vi "Message Available.vi"(8 "error in":errorcluster, 11 "VISA resource name":refnum<visa-resource-name>) -> (0 "error out":errorcluster, 2 "message available":bool, 3 "VISA resource name out":refnum<visa-resource-name>)   [LabVIEW 2019, in "Andeen-Hagerling 2700(400 firmware).lvlib"]
doc: "Poll the VISA resource to check if a message is available to read."
uses:
  Andeen-Hagerling 2700(400 firmware).lvlib
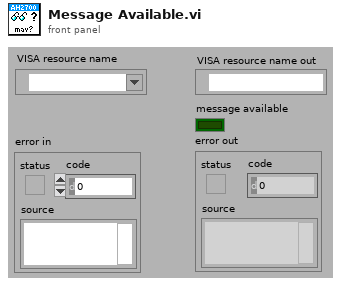
[diagram p1: front panel]
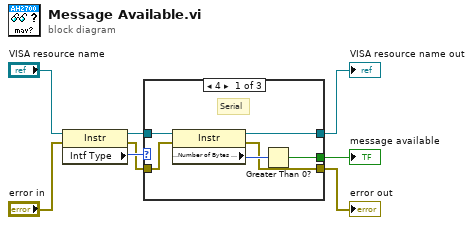
[diagram p0: block diagram]
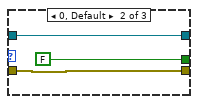
[diagram p2: hidden frame]
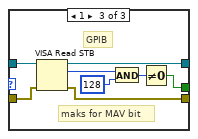
[diagram p3: hidden frame]
diagram:
  n1 = property class="Instr"(reference="VISA resource name", error in="error in") -> (reference out=w7:refnum<visa-resource-name>, error out=w2:errorcluster, "Intf Type"=w8:u16)
  n2 = case shown="4" w8 {
    tunnel: w7 -> [w14 w17 w25]
    tunnel: [w12 FALSE w20] -> w1
    tunnel: [w11 w17 w24] -> w5
    tunnel: w2 -> [w10 w15 w19]
    tunnel: [w9 w15 w18] -> w3
    frame 4 {
      # "Serial"
      n3 = property class="Instr"(reference=w14, error in=w10) -> (reference out=w11:refnum<visa-resource-name>, error out=w9:errorcluster, "Serial Settings:Number of Bytes at Serial Port"=w13:u32)
      n4 = Greater Than 0?(x=w13) -> (x > 0?=w12:bool)
    }
    frame 0, Default {
    }
    frame 1 {
      # "GPIB"
      # "maks for MAV bit"
      n5 = VISA Read STB(8:w19, 11:w25) -> (0:w18:errorcluster, 2:w23:u16, 3:w24:refnum<visa-resource-name>)
      n6 = And(x=w23, y=u16 128) -> (x .and. y?=w21:u16)
      n7 = Not Equal To 0?(x=w21) -> (x != 0?=w20:bool)
    }
  }
  "VISA resource name out" <- w5
  "error out" <- w3
  "message available" <- w1
